vi "VI defining Suite.vi"   [LabVIEW 2013, in "Unit Tests for Runner.lvclass"]
uses:
  Unit Tests for Runner.lvclass
  classes/Test Suite/Test Suite.lvclass
  classes/Test/Test.lvclass
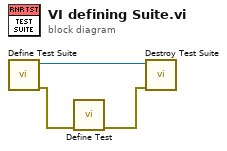
[diagram p0: block diagram]
diagram:
  n1 = call "Define Test Suite.vi"() -> ("error out"=w3:errorcluster, "Test Suite"=w1:refnum<class "Test Suite.lvclass">)  [unwired: 10 in]
  n2 = call "Define Test.vi"("error in (no error)"=w3) -> ("error out"=w2:errorcluster)  [unwired: 10 in]
  n3 = call-dynamic "Destroy Test Suite.vi"("error in (no error)"=w2, "Test Suite in"=w1) -> ()  [unwired: 9 in, 1 out]
